vi "getSb.vi"(8 "传感器索引":i32=1, 9 "检定次数":i32=1, 10 "压力点个数":i32, 11 "数据":string[][](array[string])) -> (3 "周期稳定性":dbl[](array[numeric]))   [LabVIEW 2017]
uses:
  e8dbe202-6b18-43c7-b9bc-53c255b5149f.vi
  <vilib>/Array/Sort 2D Array - Pop Stack.vi
  <vilib>/Array/Sort 2D Array - Push Stack.vi
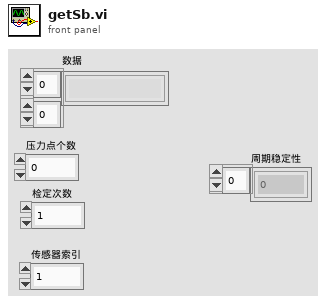
[diagram p1: front panel]
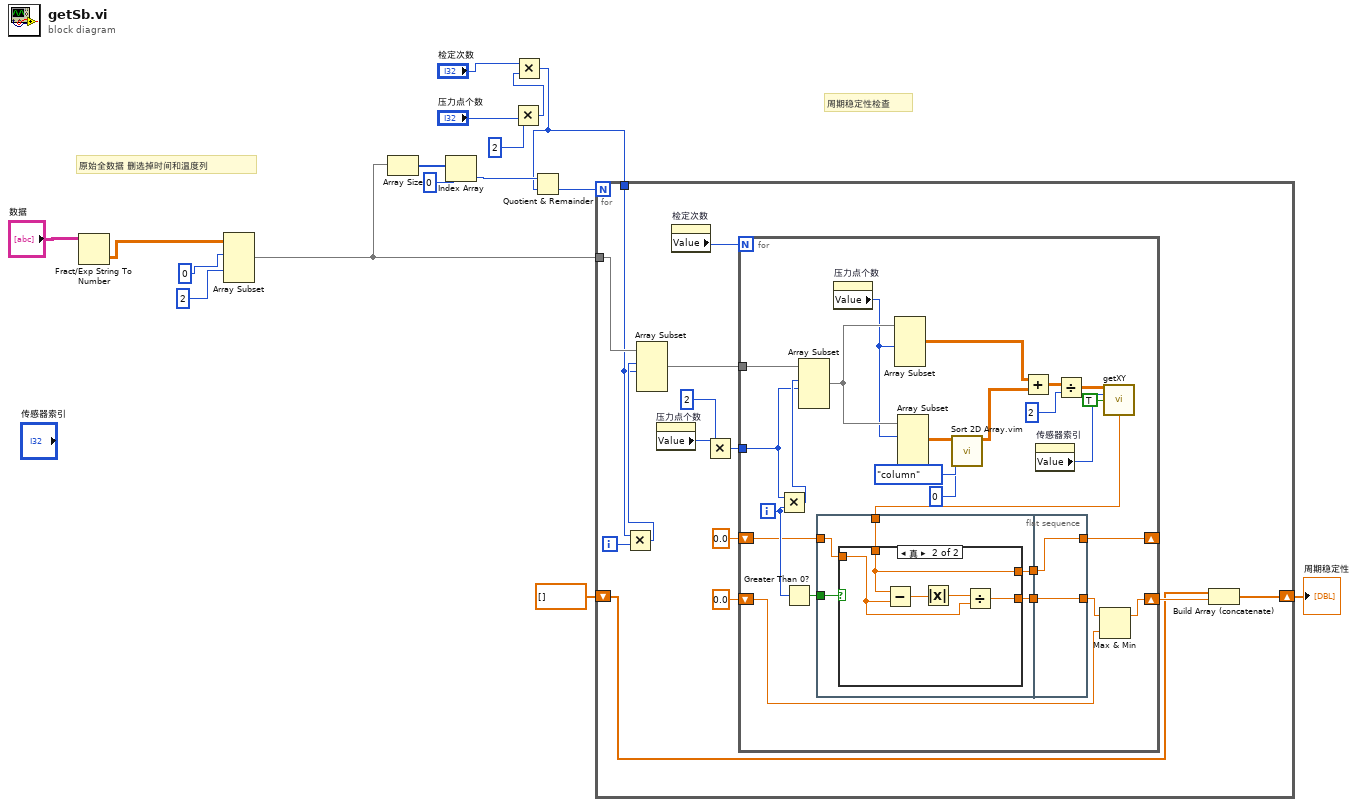
[diagram p0: block diagram]
diagram:
  # "原始全数据 删选掉时间和温度列"
  # "周期稳定性检查"
  n1 = Fract/Exp String To Number(string="数据") -> (number=w6:dbl[][])  [unwired: 3 in, 1 out]
  n2 = Array Subset(array=w6, index (row)=0 ("长度"), index (col)=2 ("索引")) -> (w4:dbl[][])  [unwired: 2 in]
  n3 = Array Size(array=w4) -> (size(s)=w12:i32[])
  n4 = Index Array(array=w12, index=0 ("索引")) -> (element=w10:i32)
  n5 = Multiply(x=2, y="压力点个数") -> (x*y=w8:i32)
  n6 = Multiply(x="检定次数", y=w8) -> (x*y=w3:i32)
  n7 = Quotient & Remainder(x=w10, y=w3) -> (floor(x/y)=w5:i32)  [unwired: 1 out]
  n8 = for {
    N: w5 -> [_]
    tunnel: w4 -> [w30]
    tunnel: w3 -> [w27]
    shift-right: [w18] -> w1
    shift-left: dbl[] [] -> [w17]
    i -> [w29]
    n9 = Multiply(x=w27, y=w29) -> (x*y=w28:i32)
    n10 = Array Subset(array=w30, index (row)=w28, length (row)=w27) -> (w25:dbl[][])  [unwired: 2 in]
    n11 = property on="压力点个数" class="DigNum (严格)"() -> ("Value"=w24:i32)  [unwired: 2 in, 2 out]
    n12 = property on="检定次数" class="DigNum (严格)"() -> ("Value"=w26:i32)  [unwired: 2 in, 2 out]
    n13 = Multiply(x=w24, y=2) -> (x*y=w22:i32)
    n14 = for {
      N: w26 -> [_]
      tunnel: w25 -> [w55]
      tunnel: w22 -> [w53]
      shift-right: [w34] -> _
      shift-left: 0.0 ("slope") -> [w37]
      shift-right: [w31] -> w19
      shift-left: 0.0 -> [w32]
      i -> [w39]
      n15 = Multiply(x=w53, y=w39) -> (x*y=w54:i32)
      n16 = Greater Than 0?(x=w39) -> (x > 0?=w40:bool)
      n17 = Array Subset(array=w55, index (row)=w54, length (row)=w53) -> (w52:dbl[][])  [unwired: 2 in]
      n18 = flat-sequence {
        tunnel: w40 -> [w60]
        tunnel: w38 -> [w59]
        tunnel: w37 -> [w58]
        tunnel: [w57] -> w36
        tunnel: [w56] -> w35
        tunnel: [w68] -> w33
        tunnel: w36 -> [w68]
        tunnel: w35 -> [w67]
        tunnel: [w67] -> w34
        frame #0 {
          n19 = case shown="真" w60 {
            tunnel: w59 -> [w61 w62]
            tunnel: w58 -> [_ w64]
            tunnel: [_ w63] -> w57
            tunnel: [w61 w62] -> w56
            frame False {
            }
            frame True {
              n20 = Subtract(x=w62, y=w64) -> (x-y=w66:dbl)
              n21 = Absolute Value(x=w66) -> (abs(x)=w65:dbl)
              n22 = Divide(x=w65, y=w64) -> (x/y=w63:dbl)
            }
          }
        }
        frame #1 {
        }
      }
      n23 = property on="压力点个数" class="DigNum (严格)"() -> ("Value"=w51:i32)  [unwired: 2 in, 2 out]
      n24 = Array Subset(array=w52, length (row)=w51) -> (w47:dbl[][])  [unwired: 3 in]
      n25 = Array Subset(array=w52, index (row)=w51) -> (w50:dbl[][])  [unwired: 3 in]
      n26 = call "Sort 2D Array.vim"("index"=0, "dimension to index (column)"=enum16{"column", "row"}."column", "2D array"=w50) -> ("sorted 2D array"=w46:dbl[][])  [unwired: 7 in, 1 out]
      n27 = Add(x=w47, y=w46) -> (x+y=w45:dbl[][])
      n28 = property on="传感器索引" class="DigNum (严格)"() -> ("Value"=w42:i32)  [unwired: 2 in, 2 out]
      n29 = Divide(x=w45, y=2) -> (x/y=w43:dbl[][])
      n30 = Max & Min(x=w33, y=w32) -> (max(x,y)=w31:dbl)  [unwired: 1 out]
      n31 = call "getXY.vi"("数据"=w43, "传感器索引"=w42, "是否需要计算拟合曲线"=TRUE) -> ("slope"=w38:dbl)  [unwired: 5 in, 7 out]
    }
    n32 = Build Array (concatenate)(w17, w19) -> (w18:dbl[])
  }
  "周期稳定性" <- w1
